vi "ReloadSession.vi"(8 "error in (no error)":errorcluster, 11 "session id in":i32) -> (0 "error out":errorcluster, 2 "ReloadSession":bool, 3 "session id out":i32)   [LabVIEW 2018, in "libonnx_wrapper.lvlib"]
doc: "/**\n * @brief Перезагрузить сессию по сохранённому пути\n * \n * Восстанавливает сессию после вызова UnloadSession. Модель загружается заново\n * из файла, путь к которому был сохранён при создании сессии.\n * \n * @param sessionId [IN] ID сессии для перезагрузки\n * \n * @return int32: 0 при успешной загрузке\n * @return int32: -1 если сессия не найдена или путь не сохранён\n * \n * @note Требует предварительного вызова CreateSession\n * @note Полезно для экономии памяти в долго работающих приложениях\n */\nint ReloadSession(int sessionId);"
uses:
  libonnx_wrapper.lvlib
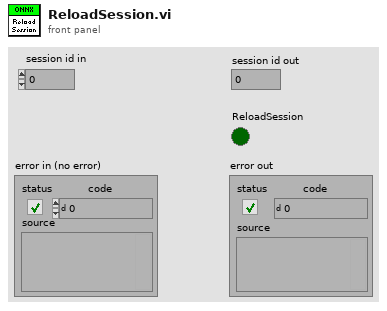
[diagram p1: front panel]
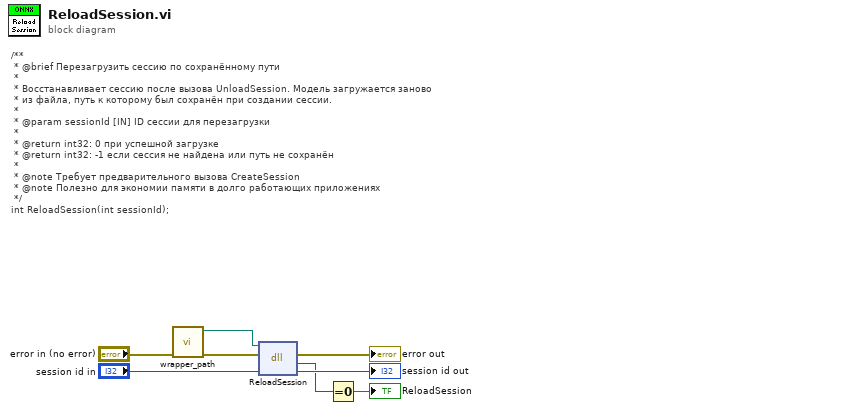
[diagram p0: block diagram]
diagram:
  # "/**\n * @brief Перезагрузить сессию по сохранённому пути\n * \n * Восстанавливает сессию после вызова UnloadSession. Модель загружается заново\n * из файла, путь к которому был сохранён при создании сессии.\n * \n * @param sessionId [IN] ID сессии для перезагрузки\n * \n * @return int32: 0 при успешной загрузке\n * @return int32: -1 если сессия не найдена или путь не сохранён\n * \n * @note Требует предварительного вызова CreateSession\n * @note Полезно для экономии памяти в долго работающих приложениях\n */\nint ReloadSession(int sessionId);"
  n1 = call "wrapper_path.vi"("error in (no error)"="error in (no error)") -> ("error out"=w6:errorcluster, "wrapper path"=w5:path)  [unwired: 9 in]
  n2 = dll-call lib="home/ivan/LabVIEWData/ONNX/Test/libonnx_wrapper/unix64/libonnx_wrapper.so" fn="ReloadSession"(path in=w5, error in=w6, "sessionId"="session id in") -> (error out=→"error out":errorcluster, "ReloadSession"=w2:i32, "sessionId"=→"session id out":i32)  [unwired: 1 in, 1 out]
  n3 = Equal To 0?(x=w2) -> (x = 0?=→"ReloadSession":bool)
